vi "DereferencingPointerToArrayOfIntegersUsingGetValueByPointer.vi"(8 "error in (no error)":errorcluster, 10 "Length":i32, 11 "Address (Pointer)":i64) -> (0 "error out":errorcluster, 3 "Value":i32[](array[numeric]))   [LabVIEW 2009, in "LabVIEWWrapper_PassingDataSampleDLL.lvlib"]
uses:
  LabVIEWWrapper_PassingDataSampleDLL.lvlib
  <vilib>/Utility/importsl/GetValueByPointer/GetValueByPointer.xnode
  <vilib>/Utility/importsl/GetValueByPointer/datatype.ctl
  Program Files (x86)/National Instruments/LabVIEW 2009/resource/lvimptsl.dll
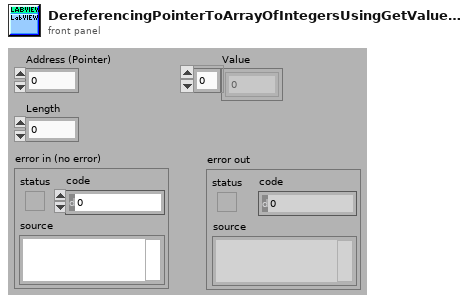
[diagram p1: front panel]
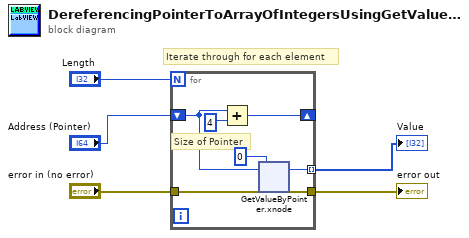
[diagram p0: block diagram]
diagram:
  # "Iterate through for each element"
  n1 = for {
    N: "Length" -> [_]
    shift-right: [w11] -> _
    shift-left: "Address (Pointer)" -> [w10]
    tunnel: [w9] -> w1 mode=indexing
    tunnel: "error in (no error)" -> [w7]
    tunnel: [w6] -> w2
    # "Size of Pointer"
    n2 = Add(x=w10, y=4) -> (x+y=w11:i64)
    n3 = xnode "GetValueByPointer.xnode"("Pointer"=w10, "InputType"=0, "ErrorIn"=w7) -> ("Output"=w9:i32, "ErrorOut"=w6:errorcluster)  [unwired: 1 in]
  }
  "error out" <- w2
  "Value" <- w1
